vi "Digital Input Test.vi"() -> ()   [LabVIEW 2020]
uses:
  <vilib>/MakerHub/LINX/Public/Peripherals/Digital/Digital Read 1 Chan.vi
  <vilib>/MakerHub/LINX/Public/Peripherals/Digital/Digital Read N Chans.vi
  <vilib>/MakerHub/LINX/Private/Local IO/LinxDigitalRead.vi
  <vilib>/MakerHub/LINX/Public/Utilities/Check Channel.vi
  <vilib>/MakerHub/LINX/Public/Utilities/Open Local.vi
  <vilib>/MakerHub/LINX/Private/Utilties/Generate Error.vi
  <vilib>/MakerHub/LINX/LMH-LINX.lvlib
panel:
  out "Array":cluster{i32, "DI ":bool, "err":bool}[](array[cluster])
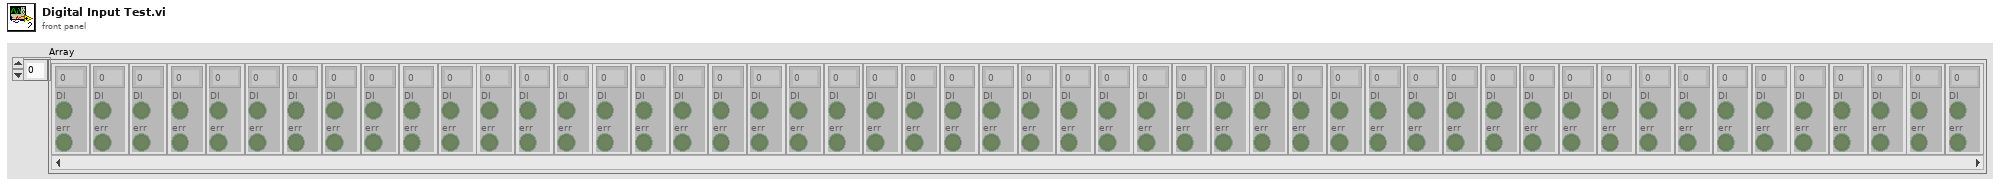
[diagram p1: front panel]
types:
  T1 = typedef "LMH-LINX.lvlib/LINX Ref.ctl" = cluster{"IO":T2, "Interface":T3, "LINX Device Config":T4}
  T2 = typedef "LMH-LINX.lvlib/Platform.ctl" = enum16{"Remote", "Local"}
  T3 = typedef "LMH-LINX.lvlib/Interface.ctl" = enum16{"Serial", "TCP"}
  T4 = typedef "LMH-LINX.lvlib/Device.lvlib/LINX Device Config.ctl" = cluster{"Interface":T3, "COM Port":refnum<visa-resource-name>, "TCP Configuration":T5, "Device Family":u8, "Device ID":u8, "Device Name":string, "TCP Ref":refnum<k5>, "Channels":T6}
  T5 = typedef "LMH-LINX.lvlib/Device.lvlib/TCP Config.ctl" = cluster{"IP Address":string, "Port":u16}
  T6 = typedef "LMH-LINX.lvlib/Channels.ctl" = cluster{"DI":u8[], "DO":u8[], "AI":u8[], "AO":u8[], "PWM":u8[], "QE":u8[], "UART":u8[], "I2C 2":u8[], "SPI":u8[], "CAN":u8[], "Servo":u8[], "AI Ref (V)":dbl, "AI Resolution (Bits)":u8, "AO Ref (V)":dbl, "AO Resolution (Bits)":u8}
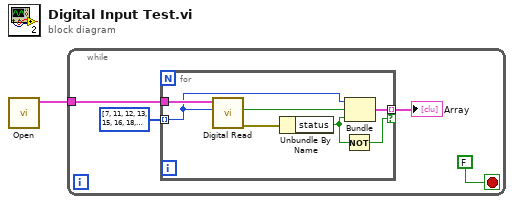
[diagram p0: block diagram]
diagram:
  n1 = call-poly <vilib>:"Open.vi"() -> ("LINX Resource"=w1:T1)  [unwired: 9 in, 2 out]
  n2 = while {
    tunnel: w1 -> [w5]
    stop <- FALSE stop-if-true
    n3 = for {
      tunnel: w5 -> [w12]
      tunnel: [w10] -> w4 mode=indexing if=w7
      tunnel: u8[] [7, 11, 12, 13, 15, 16, 18, 22, 29] ("Array 3") -> [w6] mode=indexing
      n4 = call-poly <vilib>:"Digital Read.vi"("DI Channel"=w6, "LINX Resource"=w12) -> ("Error Out"=w9:errorcluster, "DI Value"=w11:bool)  [unwired: 7 in, 1 out]
      n5 = Unbundle By Name(w9) -> ("status"=w8:bool)
      n6 = Not(x=w8) -> (.not. x?=w7:bool)
      n7 = Bundle(w6, "DI Value"=w11, "status"=w8) -> (w10:cluster{u8, "DI Value":bool, "status":bool})  [unwired: 1 in]
    }
    "Array" <- w4
  }
